vi "Serialize as XML.vi"(8 "error in (no error)":errorcluster, 11 "Reference in":refnum<class "Reference.lvclass">) -> (0 "error out":errorcluster, 2 "XML Fragment":string, 3 "Reference out":refnum<class "Reference.lvclass">)   [LabVIEW 2018, in "VILab.lvlib" / "Reference.lvclass"]
uses:
  Reference.lvclass
  Element.lvclass
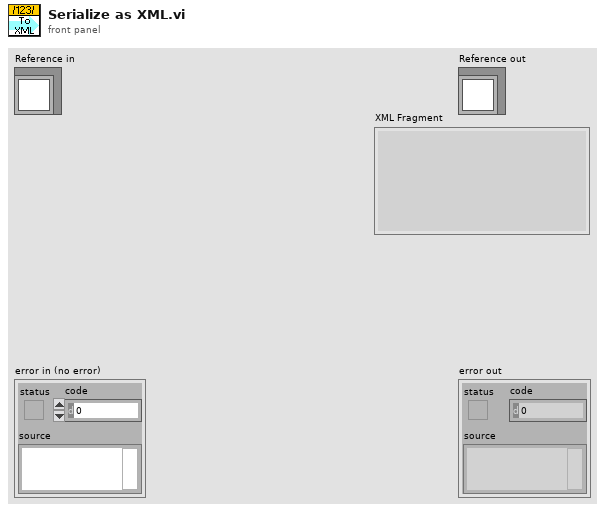
[diagram p1: front panel]
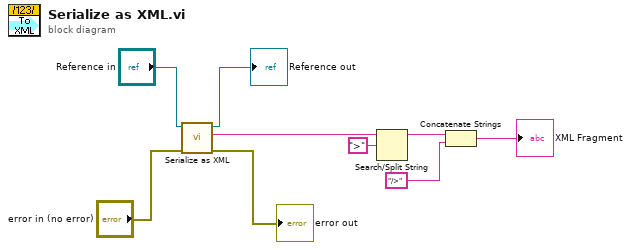
[diagram p0: block diagram]
diagram:
  n1 = call-parent "Serialize as XML.vi"("error in (no error)"="error in (no error)", "Element in"="Reference in") -> ("error out"=→"error out":errorcluster, "XML Fragment"=w5:string, "Element out"=→"Reference out":refnum<class "Reference.lvclass">)  [unwired: 7 in]
  n2 = Search/Split String(string=w5, search string/char (-)=">") -> (substring before match=w3:string)  [unwired: 1 in, 2 out]
  n3 = Concatenate Strings(w3, "/>") -> (→"XML Fragment":string)
